vi "WFS Get Instrument Info.vi"(8 "error in (no error)":errorcluster {"code" format="%.0x"}, 11 "instrument handle":refnum<visa-resource-name>) -> (0 "error out":errorcluster {"code" format="%.0x"}, 1 "Instrument Name WFS":string, 2 "Manufacturer Name":string, 3 "instrument handle out":refnum<visa-resource-name>, 4 "Serial Number WFS":string, 5 "Serial Number Cam":string)   [LabVIEW 2020]
doc: "This VI returns the following information about the opened instrument:\n- Driver Manufacturer Name\n- Instrument Name\n- Instrument Serial Number\n- Camera Serial Number"
uses:
  WFS_32.dll
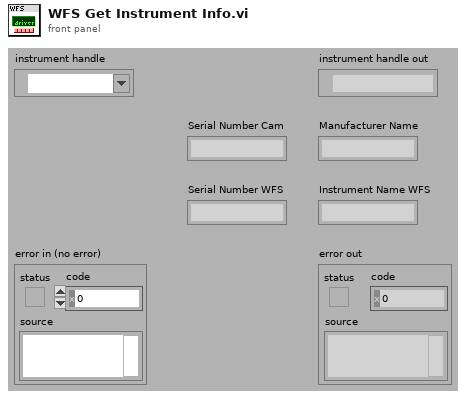
[diagram p1: front panel]
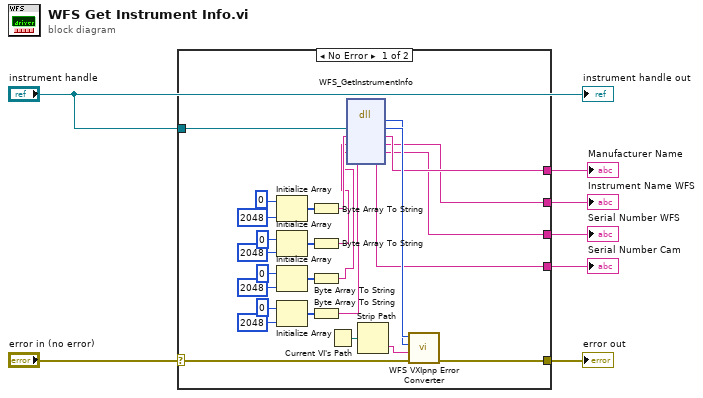
[diagram p0: block diagram]
diagram:
  n1 = case shown="No Error" "error in (no error)" {
    selector: "error in (no error)" -> [w29 w35]
    tunnel: [w28 w35] -> w7
    tunnel: "instrument handle" -> [w33 _]
    tunnel: [w23 _] -> w4
    tunnel: [w18 _] -> w3
    tunnel: [w13 _] -> w2
    tunnel: [w8 _] -> w1
    frame No Error {
      n2 = Initialize Array(u8 0 ("element"), 2048 ("dimension size")) -> (w26:u8[])
      n3 = Initialize Array(u8 0 ("element"), 2048 ("dimension size")) -> (w21:u8[])
      n4 = Initialize Array(u8 0 ("element"), 2048 ("dimension size")) -> (w16:u8[])
      n5 = Initialize Array(u8 0 ("element"), 2048 ("dimension size")) -> (w11:u8[])
      n6 = Byte Array To String(unsigned byte array=w26) -> (string=w27:string)
      n7 = Byte Array To String(unsigned byte array=w21) -> (string=w22:string)
      n8 = Byte Array To String(unsigned byte array=w16) -> (string=w17:string)
      n9 = Byte Array To String(unsigned byte array=w11) -> (string=w12:string)
      n10 = Current VI's Path() -> (path=w34:path)
      n11 = dll-call lib="WFS_*.*" fn="WFS_GetInstrumentInfo"("Instrument Handle"=w33, "Manufacturer Name"=w27, "Instrument Name WFS"=w22, "Serial Number WFS"=w17, "Serial Number Cam"=w12) -> (w31:i32, "Instrument Handle"=w32:u32, "Manufacturer Name"=w23:string, "Instrument Name WFS"=w18:string, "Serial Number WFS"=w13:string, "Serial Number Cam"=w8:string)  [unwired: 3 in, 2 out]
      n12 = Strip Path(path=w34) -> (name=w30:string)  [unwired: 1 out]
      n13 = call "WFS VXIpnp Error Converter.vi"("error in (no error)"=w29, "Name Of VI (\"\")"=w30, "CVI Error Code (0)"=w31, "instrument handle"=w32) -> ("error out"=w28:errorcluster)  [unwired: 6 in, 1 out]
    }
    frame Error {
    }
  }
  "error out" <- w7
  "Manufacturer Name" <- w4
  "Instrument Name WFS" <- w3
  "Serial Number WFS" <- w2
  "Serial Number Cam" <- w1
  "instrument handle out" <- "instrument handle"
